vi "Correlation Coefficient (Spearman).vi"(10 "Y":dbl[](array[numeric]) format="%.2f", 11 "X":dbl[](array[numeric]) format="%.2f") -> (2 "r^2":dbl format="%.7g", 3 "correlation coefficient r":dbl format="%.7g")   [LabVIEW 2017, in "NI_Gmath.lvlib"]
doc: "Computes the Spearman's rank correlation coefficient between input sequences <B>X</B> and <B>Y</B>."
uses:
  NI_Gmath.lvlib
  NI_AALPro.lvlib
panel:
  # "Correlation Coefficient \n(Spearman Rank-Order)"
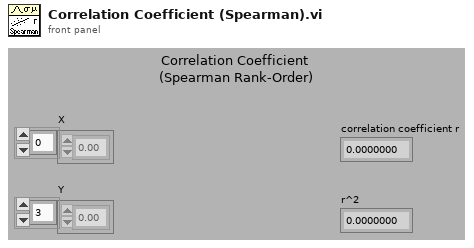
[diagram p1: front panel]
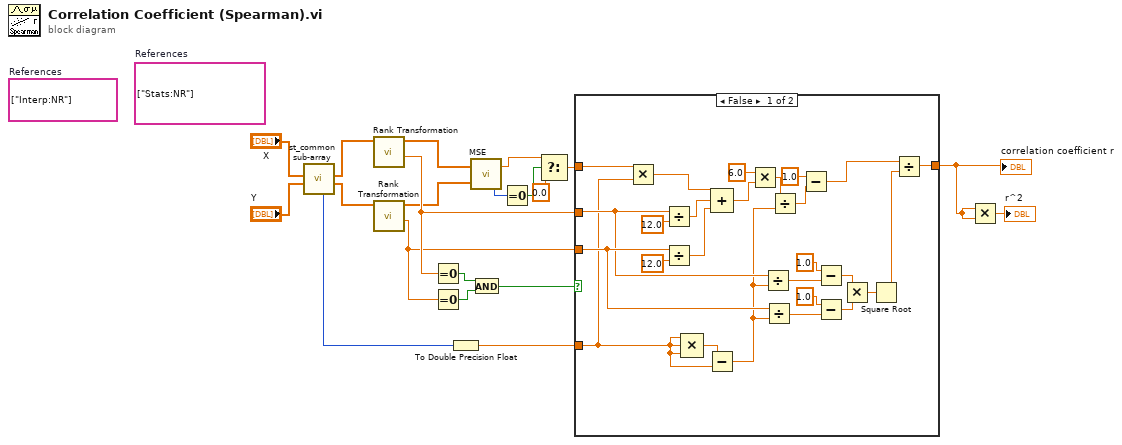
[diagram p0: block diagram]
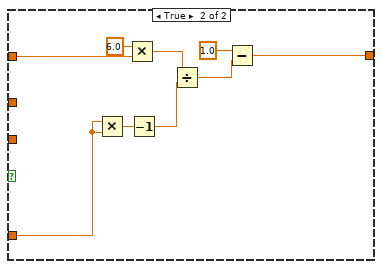
[diagram p2: hidden frame]
diagram:
  (unwired) string[] ["Stats:NR"]  # References
  (unwired) string[] ["Interp:NR"]  # References
  n1 = call "st_common sub-array.vi"(9:"array 1 in"="Y", 10:"array 1 in"="X") -> (1:"array 1 out"=w19:dbl[], 2:"array 1 out"=w20:dbl[], "size"=w18:i32)  [unwired: 7 in]
  n2 = call "Rank Transformation.vi"("x"=w20) -> ("tsum - measure of ties"=w13:dbl, "rank order x"=w3:dbl[])  [unwired: 9 in]
  n3 = call "Rank Transformation.vi"("x"=w19) -> ("tsum - measure of ties"=w12:dbl, "rank order x"=w2:dbl[])  [unwired: 9 in]
  n4 = Equal To 0?(x=w13) -> (x = 0?=w16:bool)
  n5 = Equal To 0?(x=w12) -> (x = 0?=w15:bool)
  n6 = To Double Precision Float(number=w18) -> (double precision float=w11:dbl)
  n7 = call "MSE.vi"("X Values"=w2, "Y Values"=w3) -> ("error"=w10:i32, "mse"=w8:dbl)
  n8 = And(x=w16, y=w15) -> (x .and. y?=w14:bool)
  n9 = Equal To 0?(x=w10) -> (x = 0?=w9:bool)
  n10 = Select(t=w8, s=w9, f=0.0) -> (s? t:f=w7:dbl)
  n11 = case shown="False" w14 {
    tunnel: w11 -> [w21 w53]
    tunnel: [w24 w50] -> w1
    tunnel: w7 -> [w39 w47]
    tunnel: w13 -> [w33 _]
    tunnel: w12 -> [w34 _]
    frame False {
      n12 = Multiply(x=w39, y=w21) -> (x*y=w38:dbl)
      n13 = Divide(x=w33, y=12.0 ("x")) -> (x/y=w40:dbl)
      n14 = Divide(x=w34, y=12.0 ("x")) -> (x/y=w41:dbl)
      n15 = Compound Arithmetic op=MULTIPLY(w21, w21, w21) -> (w36:dbl)
      n16 = Subtract(x=w36, y=w21) -> (x-y=w32:dbl)
      n17 = Compound Arithmetic op=ADD(w38, w40, w41) -> (w37:dbl)
      n18 = Multiply(x=6.0, y=w37) -> (x*y=w45:dbl)
      n19 = Divide(x=w33, y=w32) -> (x/y=w30:dbl)
      n20 = Divide(x=w34, y=w32) -> (x/y=w28:dbl)
      n21 = Divide(x=w45, y=w32) -> (x/y=w44:dbl)
      n22 = Subtract(x=1.0, y=w44) -> (x-y=w23:dbl)
      n23 = Subtract(x=1.0, y=w30) -> (x-y=w27:dbl)
      n24 = Subtract(x=1.0, y=w28) -> (x-y=w26:dbl)
      n25 = Multiply(x=w27, y=w26) -> (x*y=w25:dbl)
      n26 = Square Root(x=w25) -> (sqrt(x)=w22:dbl)
      n27 = Divide(x=w23, y=w22) -> (x/y=w24:dbl)
    }
    frame True {
      n28 = Multiply(x=w53, y=w53) -> (x*y=w49:dbl)
      n29 = Multiply(x=6.0, y=w47) -> (x*y=w52:dbl)
      n30 = Decrement(x=w49) -> (x-1=w48:dbl)
      n31 = Divide(x=w52, y=w48) -> (x/y=w51:dbl)
      n32 = Subtract(x=1.0, y=w51) -> (x-y=w50:dbl)
    }
  }
  "correlation coefficient r" <- w1
  n33 = Multiply(x=w1, y=w1) -> (x*y=→"r^2":dbl)
